vi "offset cal.vi"(8 "error in (no error)":errorcluster, 9 "read_dl950":string, 10 "index low":i32, 11 "index level":i32) -> (0 "error out":errorcluster, 3 "output array":dbl[](array[numeric]))   [LabVIEW 2019]
panel:
  out "array":dbl[](array[numeric])
  out "read_dl950":string
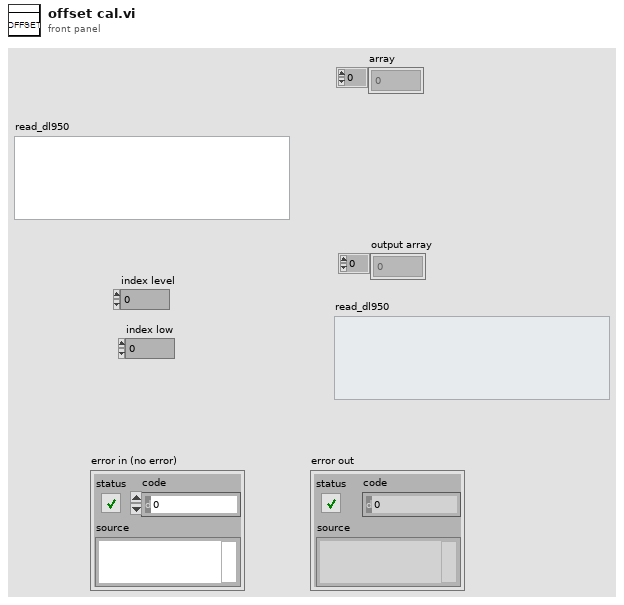
[diagram p1: front panel]
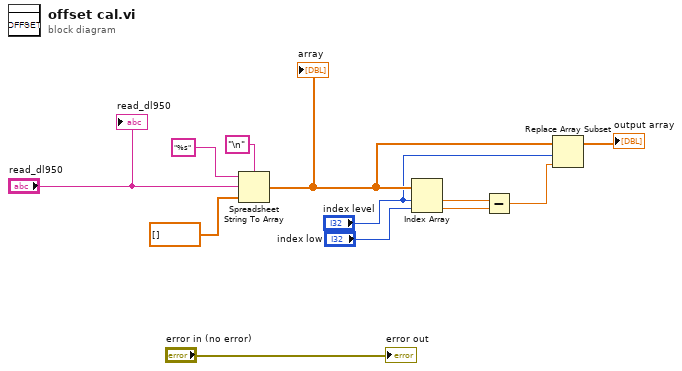
[diagram p0: block diagram]
diagram:
  n1 = Spreadsheet String To Array(delimiter (Tab)="\n", format string="%s", spreadsheet string="read_dl950", array type (2D Dbl)=dbl[] []) -> (array=w5:dbl[])
  "array" <- w5
  n2 = Index Array(array=w5, index #1="index level", index #2="index low") -> (element #1=w7:dbl, element #2=w6:dbl)
  n3 = Subtract(x=w7, y=w6) -> (x-y=w3:dbl)
  n4 = Replace Array Subset(array=w5, new element=w3, index="index level") -> (→"output array":dbl[])
  "read_dl950" <- "read_dl950"
  "error out" <- "error in (no error)"
